vi "WebDAV Daten speichern auf PC.vi"(7 "IP Adresse":string, 8 "error in":errorcluster, 10 "Dateinamen":string[](array[string]), 11 "Pfad PC":path caption="Lokaler Pfad") -> (0 "error out":errorcluster, 2 "ohne Fehler":bool)   [LabVIEW 2020, in "Backup.lvlib"]
uses:
  Backup.lvlib
  <vilib>/WebDAVClient/Simple Get File.vi
  <vilib>/FTP/NI_FTP.lvlib
  <vilib>/WebDAVClient/NI_WebDAV.lvlib
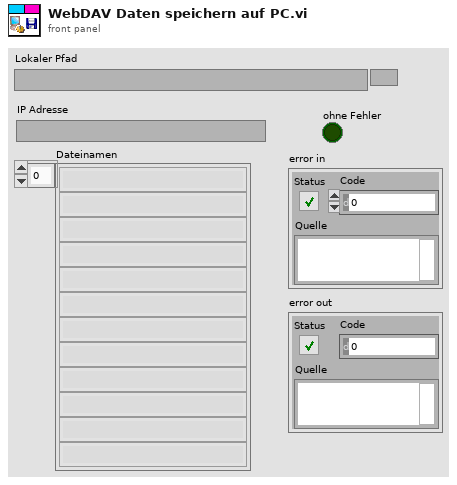
[diagram p1: front panel]
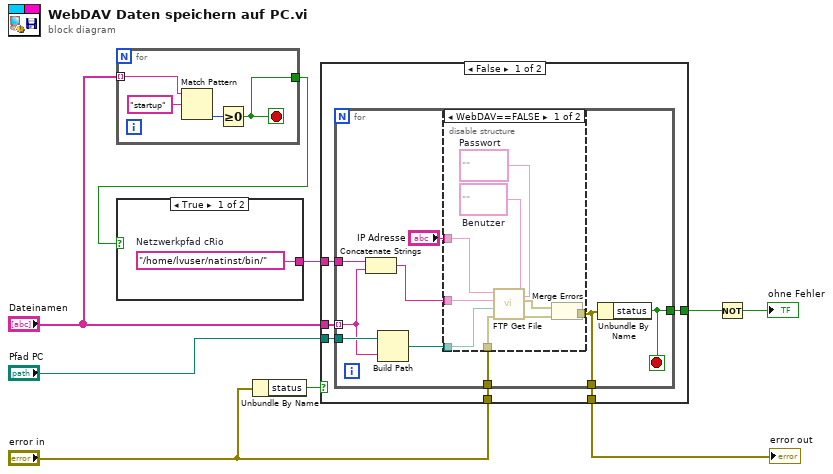
[diagram p0: block diagram]
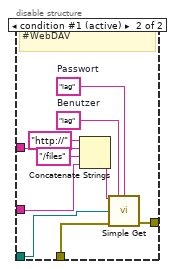
[diagram p2: hidden frame]
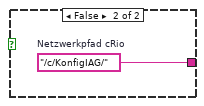
[diagram p4: hidden frame]
diagram:
  n1 = for {
    tunnel: "Dateinamen" -> [w11] mode=indexing
    tunnel: [w10] -> w9
    stop <- w10 stop-if-true
    n2 = Match Pattern(string=w11, regular expression="startup" ("Regulärer Ausdruck")) -> (offset past match=w13:i32)  [unwired: 1 in, 3 out]
    n3 = Greater Or Equal To 0?(x=w13) -> (x >= 0?=w10:bool)
  }
  n4 = case shown="True" w9 {
    tunnel: [w14 w15] -> w7
    frame True {
      w14 = "/home/lvuser/natinst/bin/"  # Netzwerkpfad cRio
    }
    frame False {
      w15 = "/c/KonfigIAG/"  # Netzwerkpfad cRio
    }
  }
  n5 = Unbundle By Name("error in") -> ("status"=w4:bool)
  n6 = case shown="False" w4 {
    selector: w4 -> [_ w50]
    tunnel: "Dateinamen" -> [w21 _]
    tunnel: w7 -> [w20 _]
    tunnel: "Pfad PC" -> [w19 _]
    tunnel: [w18 w51] -> w3
    tunnel: [w16 w50] -> w2
    tunnel: "error in" -> [w17 w51]
    frame False {
      n7 = for {
        tunnel: w19 -> [w28]
        tunnel: w20 -> [w30]
        tunnel: w21 -> [w27] mode=indexing
        tunnel: [w23] -> w16
        tunnel: w17 -> [w25]
        tunnel: [w24] -> w18
        stop <- w23 stop-if-true
        n8 = Concatenate Strings(w30, w27) -> (w29:string)
        n9 = Build Path(base path=w28, name or relative path=w27) -> (appended path=w26:path)
        n10 = disable-structure shown="WebDAV==FALSE" {
          disable-tunnel: w29 -> [w35 w46]
          disable-tunnel: w26 -> [w34 w40]
          disable-tunnel: w25 -> [w33 w41]
          disable-tunnel: [w32 w45] -> w24
          disable-tunnel: "IP Adresse" -> [w31 w47]
          frame condition #0 {
            w38 = ""  # Passwort
            w39 = ""  # Benutzer
            n11 = call <vilib>:"FTP Get File.vi"("password"=w38, "user"=w39, "error in (no error)"=w33, "local path"=w34, "remote path"=w35, "host"=w31) -> ("error out"=w37:errorcluster, "file error"=w36:errorcluster)  [unwired: 4 in]
            n12 = Merge Errors(w36, w37) -> (w32:errorcluster)
          }
          frame condition #1 (active) {
            w44 = "iag"  # Passwort
            w43 = "iag"  # Benutzer
            # "#WebDAV"
            n13 = Concatenate Strings("http://" ("String"), w47, "/files" ("String"), w46) -> (w42:string)
            n14 = call-poly <vilib>:"Simple Get.vi"("remote file uri"=w42, "username"=w43, "password"=w44, "local file path"=w40, "error in (no error)"=w41) -> ("error out"=w45:errorcluster)  [unwired: 9 in, 1 out]
          }
        }
        n15 = Unbundle By Name(w24) -> ("status"=w23:bool)
      }
    }
    frame True {
    }
  }
  "error out" <- w3
  n16 = Not(x=w2) -> (.not. x?=→"ohne Fehler":bool)
